vi "Write Tags.vi"(8 "error in (no error)":errorcluster, 11 "State in":T1={"State"=enum."Idle", "Start Time"=timestamp(0 s since 1904-01-01), "Configuration"={"DAQmx Task Name"="", "Output Channel Name"=0, "Time On (Sec)"=0.0, "Time Off (Sec)"=0.0}, "Current Time"=timestamp(0 s since 1904-01-01), "First Iteration"=FALSE, "Data"={"D-O State"=0}, "Process Name"="", "Output Error"=FALSE, "Log Started"=FALSE} {"Data"."D-O State" items=["Default", "On", "Off", "Not Initialized"]}) -> (0 "error out":errorcluster, 3 "State out":T1={"State"=enum."Idle", "Start Time"=timestamp(0 s since 1904-01-01), "Configuration"={"DAQmx Task Name"="", "Output Channel Name"=0, "Time On (Sec)"=0.0, "Time Off (Sec)"=0.0}, "Current Time"=timestamp(0 s since 1904-01-01), "First Iteration"=FALSE, "Data"={"D-O State"=0}, "Process Name"="", "Output Error"=FALSE, "Log Started"=FALSE} {"Data"."D-O State" items=["Default", "On", "Off", "Not Initialized"]})   [LabVIEW 2018, in "D-O Module.lvlib" / "D-O Module Engine.lvlib"]
uses:
  D-O Module Engine.lvlib
  Shared Variables/Dynamic Shared Variables.lvlib
  Tag VIs/Tag FGV Operation Enum.ctl
  State Enum.ctl
  D-O Module Settings Cluster.ctl
  D-O Module.lvlib
  State Cluster.ctl
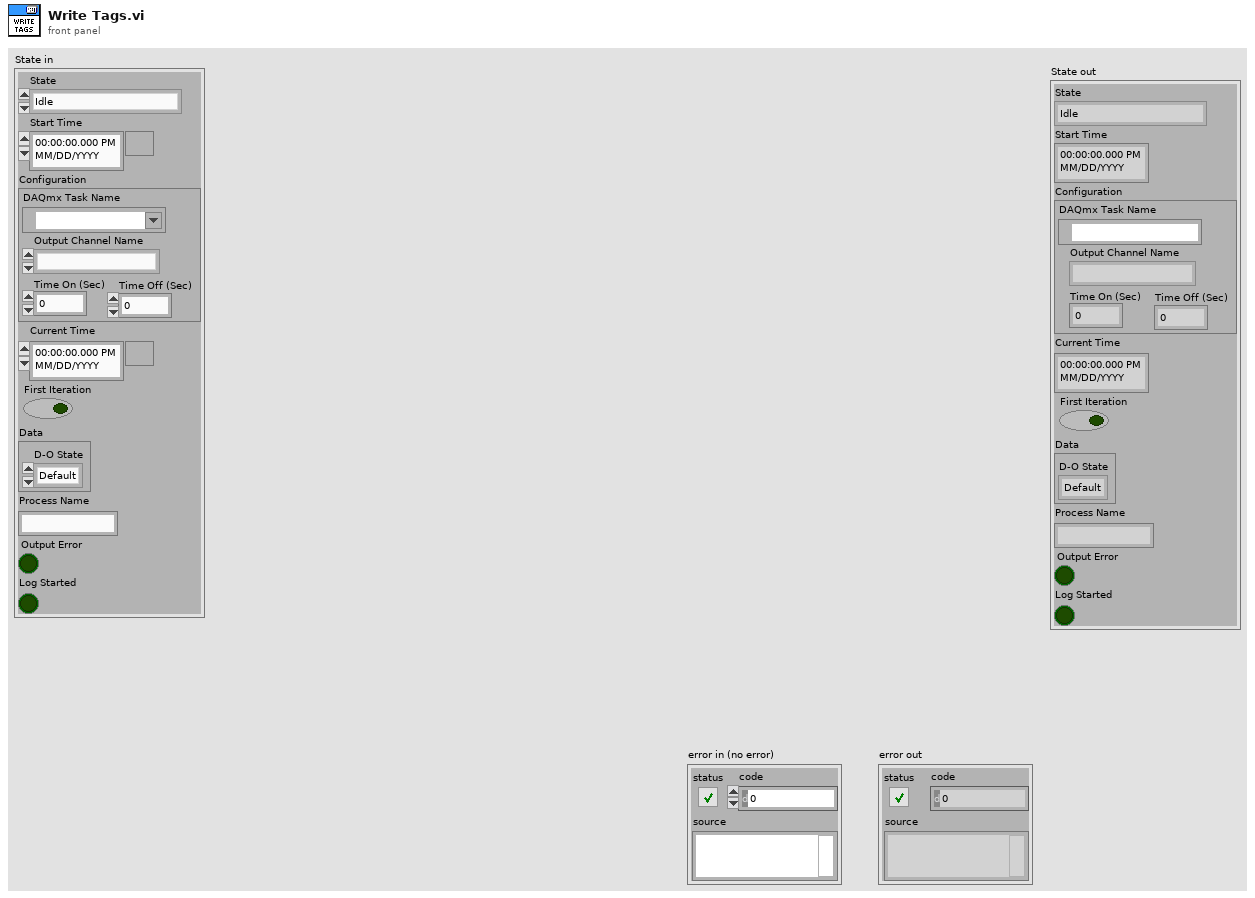
[diagram p1: front panel]
types:
  T1 = typedef "D-O Module.lvlib/D-O Module Engine.lvlib/State Cluster.ctl" = cluster{"State":T2, "Start Time":timestamp, "Configuration":T3, "Current Time":timestamp, "First Iteration":bool, "Data":cluster{"D-O State":u16}, "Process Name":string, "Output Error":bool, "Log Started":bool}
  T2 = typedef "D-O Module.lvlib/D-O Module Engine.lvlib/State Enum.ctl" = enum16{"Measuring", "Idle", "Paused"}
  T3 = typedef "D-O Module.lvlib/D-O Module Settings Cluster.ctl" = cluster{"DAQmx Task Name":refnum<k21>, "Output Channel Name":u16, "Time On (Sec)":dbl, "Time Off (Sec)":dbl}
  T4 = typedef "Tag FGV Operation Enum.ctl" = enum16{"Init", "Set Notification Queue", "Create Tag", "Write Tag (Numeric)", "Write Tag (Boolean)", "Read All Tags", "Read One Tag", "Delete Tag Category", "Set Alarm Parameters (Numeric)", "Set Alarm Parameters (Boolean)", "Enable All Alarms", "Disable All Alarms", "Delete All Tags", "Read Alarms", "Ack Alarm"}
  T5 = typedef "D-O Module.lvlib/D-O Module Tag Names Cluster.ctl" = cluster{"D-O Status":string, "Output Device Tag":string}
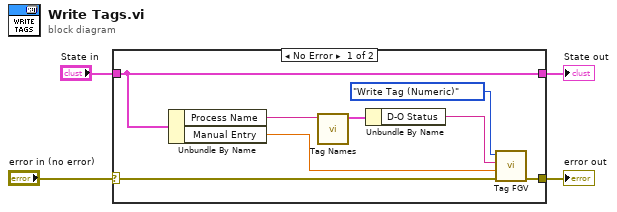
[diagram p0: block diagram]
diagram:
  n1 = case shown="No Error" "error in (no error)" {
    selector: "error in (no error)" -> [w6 w14]
    tunnel: [w7 w14] -> w3
    tunnel: "State in" -> [w10 w13]
    tunnel: [w10 w13] -> w1
    frame No Error {
      n2 = Unbundle By Name(w10) -> ("Process Name"=w12:string, "Manual Entry"=w5:dbl)
      n3 = call "Tag Names.vi"("Process Name"=w12) -> ("Pump Module Tag Names"=w9:T5)  [unwired: 8 in, 2 out]
      n4 = Unbundle By Name(w9) -> ("D-O Status"=w8:string)
      n5 = call "Tag FGV.vi"("error in (no error)"=w6, "Data"=w5, "Tag Name"=w8, "Operation"=Tag_FGV_Operation_Enum."Write Tag (Numeric)") -> ("error out"=w7:errorcluster)  [unwired: 2 in, 5 out]
    }
    frame Error {
    }
  }
  "error out" <- w3
  "State out" <- w1
